vi "웹서버 수정 버전 1.vi"() -> ()   [LabVIEW 2019]
uses:
  <vilib>/httpClient/ClientHandle.ctl
  <vilib>/DAQmx/read.llb/DAQmx Read (Digital 1D Bool NChan 1Samp 1Line).vi
  <vilib>/DAQmx/read.llb/DAQmx Read (Analog 1D DBL 1Chan NSamp).vi
  <vilib>/Analysis/baseanly.llb/Mean (DBL).vi
  <vilib>/DAQmx/create/channels.llb/DAQmx Create Channel (DI-Digital Input).vi
  <vilib>/DAQmx/configure/timing.llb/DAQmx Timing (Sample Clock).vi
  <vilib>/DAQmx/create/channels.llb/DAQmx Create Channel (AI-Temperature-Thermocouple).vi
  <vilib>/httpClient/PUTBuffer.vi
  <vilib>/DAQmx/miscellaneous.llb/DAQmx Fill In Error Info.vi
  <vilib>/httpClient/LabVIEWHTTPClient.lvlib
  <vilib>/Analysis/NI_AALBase.lvlib
panel:
  out "y 3":u32
  out "y 2":u32
  out "F포맷 문자열":string[](array[string])
  out "data":bool[](array[boolean]) caption="데이터"
  out "headers 4":string caption="연결확인 메세지 출력"
  out "body 4":string caption="웹서버에 입력된 문자열"
  out "참조 번호 출력 2":T1 caption="client handle out"
  out "10진수 문자열":string[](array[string])
  in  "정지 2":bool
  in  "lines":tag caption="라인"
  in  "thermocouple type":i32(ring)=10072 caption="열전쌍 타입" items=["J"=10072, "K"=10073, "N"=10077, "R"=10082, "S"=10085, "T"=10086, "B"=10047, "E"=10055]
  in  "physical channels":tag caption="물리적 채널"
  out "숫자형":i32
  in  "불리언":bool
  out "y":u32
  out "headers 3":string caption="연결확인 메세지 출력"
  out "body 3":string caption="웹서버에 입력된 문자열"
  in  "참조 번호 입력":T1 caption="client handle out"
  out "참조 번호 출력":T1 caption="client handle out"
  out "error out":errorcluster caption="에러 출력"
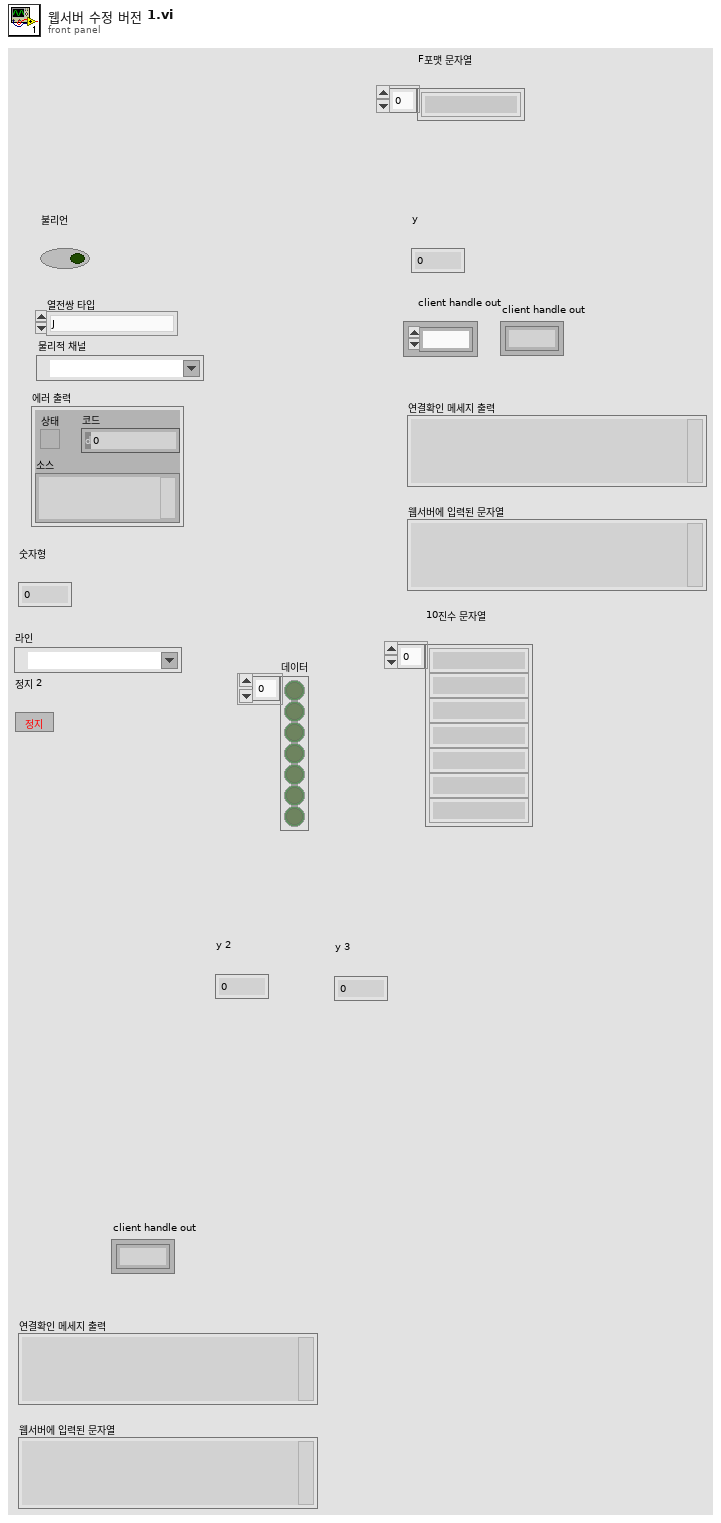
[diagram p1: front panel]
types:
  T1 = typedef "LabVIEWHTTPClient.lvlib/ClientHandle.ctl" = refnum<k1>
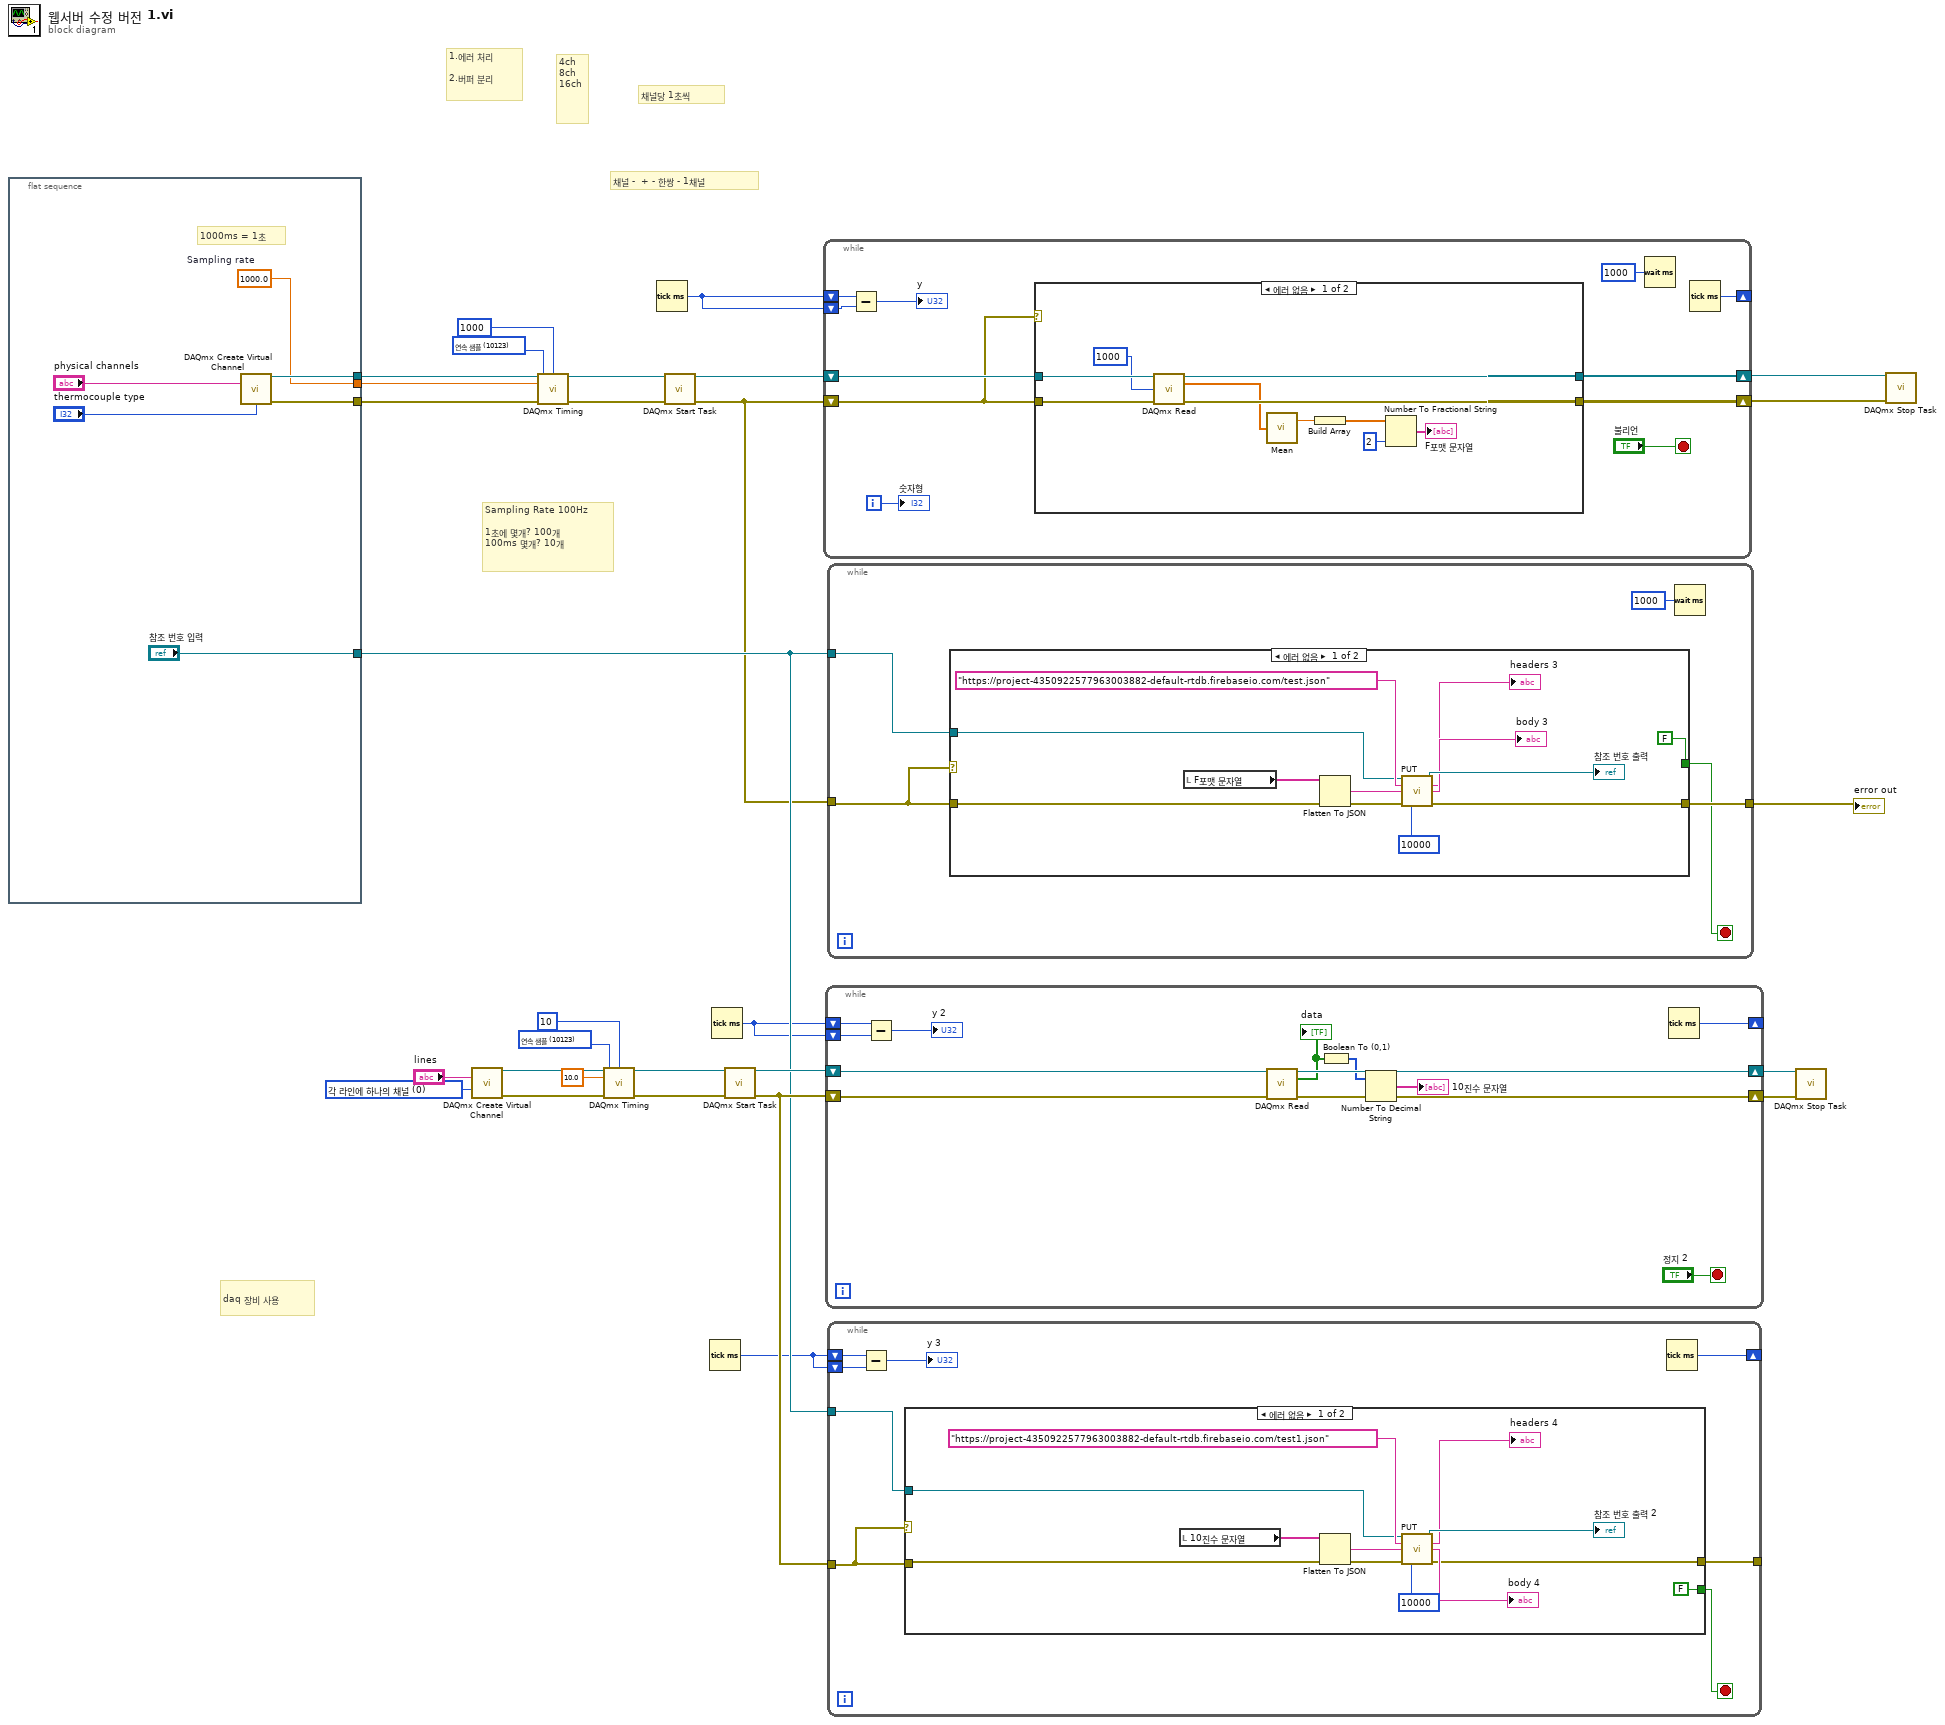
[diagram p0: block diagram]
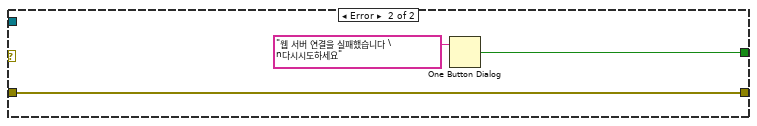
[diagram p2: hidden frame]
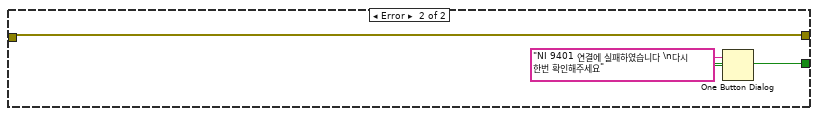
[diagram p4: hidden frame]
diagram:
  w20 = 10123 items=["유한 샘플"=10178, "연속 샘플"=10123, "하드웨어 타이밍에 의한 단일 포인트"=12522] ("sample mode")
  w21 = 0 items=["각 라인에 하나의 채널", "모든 라인에 하나의 채널"] ("line grouping")
  w23 = 10123 items=["유한 샘플"=10178, "연속 샘플"=10123, "하드웨어 타이밍에 의한 단일 포인트"=12522] ("sample mode")
  # "daq 장비 사용"
  # "1.에러 처리 \n\n2.버퍼 분리"
  # "채널 -  + - 한쌍 - 1채널"
  # "채널당 1초씩"
  # "4ch\n8ch\n16ch"
  # "Sampling Rate 100Hz\n\n1초에 몇개? 100개\n100ms 몇개? 10개"
  n1 = flat-sequence {
    tunnel: [w33] -> w29
    tunnel: [w32] -> w27
    tunnel: [w31] -> w24
    tunnel: ["참조 번호 입력"] -> w14
    frame #0 {
      w31 = 1000.0  # Sampling rate
      # "1000ms = 1초"
      n2 = call-poly <vilib>:"DAQmx Create Virtual Channel.vi"("physical channels"="physical channels", "thermocouple type"="thermocouple type") -> ("task out"=w33:refnum<k21>, "error out"=w32:errorcluster)  [unwired: 12 in]
    }
  }
  n3 = call-poly <vilib>:"DAQmx Create Virtual Channel.vi"("lines"="lines", "line grouping"=w21) -> ("task out"=w1:refnum<k21>, "error out"=w18:errorcluster)  [unwired: 12 in]
  n4 = call-poly <vilib>:"DAQmx Timing.vi"("task/channels in"=w29, "sample mode"=w23, "samples per channel"=1000, "rate"=w24, "error in"=w27) -> ("task out"=w28:refnum<k21>, "error out"=w26:errorcluster)  [unwired: 9 in]
  n5 = call-poly <vilib>:"DAQmx Timing.vi"("task/channels in"=w1, "sample mode"=w20, "samples per channel"=10, "rate"=10.0, "error in"=w18) -> ("task out"=w17:refnum<k21>, "error out"=w16:errorcluster)  [unwired: 9 in]
  n6 = Tick Count (ms)() -> (millisecond timer value=w6:u32)
  n7 = call <vilib>:"DAQmx Start Task.vi"("task/channels in"=w28, "error in"=w26) -> ("task out"=w7:refnum<k21>, "error out"=w5:errorcluster)  [unwired: 12 in]
  n8 = Tick Count (ms)() -> (millisecond timer value=w2:u32)
  n9 = Tick Count (ms)() -> (millisecond timer value=w3:u32)
  n10 = call <vilib>:"DAQmx Start Task.vi"("task/channels in"=w17, "error in"=w16) -> ("task out"=w22:refnum<k21>, "error out"=w15:errorcluster)  [unwired: 12 in]
  n11 = while {
    shift-right: [w45] -> w9
    shift-left: w7 -> [w46]
    shift-right: [w44] -> w8
    shift-left: w5 -> [w36]
    shift-right: [w41] -> _
    shift-left: w6 -> [w40]
    shift-left: w6 -> [w39]
    i -> [w43]
    stop <- "불리언" stop-if-true
    n12 = Subtract(x=w40, y=w39) -> (x-y=→"y":u32)
    n13 = case shown="에러 없음" w36 {
      tunnel: w46 -> [w56 w58]
      tunnel: w36 -> [w55 w57]
      tunnel: [w54 w58] -> w45
      tunnel: [w53 w57] -> w44
      frame No Error {
        n14 = call-poly <vilib>:"DAQmx Read.vi"("task/channels in"=w56, "number of samples per channel"=1000, "error in"=w55) -> ("task out"=w54:refnum<k21>, "data"=w49:dbl[], "error out"=w53:errorcluster)  [unwired: 10 in]
        n15 = call-poly <vilib>:"Mean.vi"("X"=w49) -> ("mean"=w48:dbl)  [unwired: 1 out]
        n16 = Build Array(w48) -> (w51:dbl[])
        n17 = Number To Fractional String(number=w51, precision (6)=i16 2 ("정밀도(6)")) -> (F-format string=→"F포맷 문자열":string[])  [unwired: 2 in]
      }
      frame Error {
        # "에러 발생시 재 연결 실시"
      }
    }
    n18 = Wait (ms)(milliseconds to wait=u32 1000 ("대기 시간 (ms)")) -> ()  [unwired: 1 out]
    n19 = Tick Count (ms)() -> (millisecond timer value=w41:u32)
    "숫자형" <- w43
  }
  n20 = while {
    shift-right: [w68] -> w12
    shift-left: w22 -> [w70]
    shift-right: [w67] -> w11
    shift-left: w15 -> [w69]
    shift-right: [w59] -> _
    shift-left: w3 -> [w61]
    shift-left: w3 -> [w60]
    stop <- "정지 2" stop-if-true
    n21 = Subtract(x=w61, y=w60) -> (x-y=→"y 2":u32)
    n22 = call-poly <vilib>:"DAQmx Read.vi"("task/channels in"=w70, "error in"=w69) -> ("task out"=w68:refnum<k21>, "data"=w64:bool[], "error out"=w67:errorcluster)  [unwired: 11 in]
    "data" <- w64
    n23 = Boolean To (0,1)(Boolean=w64) -> (0, 1=w63:i16[])
    n24 = Number To Decimal String(number=w63) -> (decimal integer string=→"10진수 문자열":string[])  [unwired: 1 in]
    n25 = Tick Count (ms)() -> (millisecond timer value=w59:u32)
  }
  n26 = while {
    tunnel: w5 -> [w72]
    tunnel: w14 -> [w74]
    tunnel: [w73] -> w4
    stop <- w71 stop-if-true
    n27 = case shown="에러 없음" w72 {
      tunnel: w72 -> [w80 w89]
      tunnel: w74 -> [w79 _]
      tunnel: [w78 w89] -> w73
      tunnel: [FALSE ("true") w88] -> w71
      frame No Error {
        n28 = local read "F포맷 문자열"() -> (w77:string[])
        n29 = Flatten To JSON(anything=w77, error in (no error)=w80) -> (JSON string=w84:string, 11:w83:errorcluster)  [unwired: 1 in]
        n30 = call-poly <vilib>:"PUT.vi"("client handle"=w79, "url"="https://project-4350922577963003882-default-rtdb.firebaseio.com/test.json", "buffer"=w84, "error in (no error)"=w83, "timeout (10000)"=10000) -> ("client handle out"=→"참조 번호 출력":T1, "headers"=→"headers 3":string, "body"=→"body 3":string, "error out"=w78:errorcluster)  [unwired: 7 in]
      }
      frame Error {
        n31 = One Button Dialog(message="웹 서버 연결을 실패했습니다 \n다시시도하세요" ("메시지")) -> (true=w88:bool)  [unwired: 1 in]
      }
    }
    n32 = Wait (ms)(milliseconds to wait=u32 1000 ("대기 시간 (ms)")) -> ()  [unwired: 1 out]
  }
  "error out" <- w4
  n33 = while {
    tunnel: w14 -> [w98]
    tunnel: [w97] -> _
    tunnel: w15 -> [w96]
    shift-right: [w94] -> _
    shift-left: w2 -> [w92]
    shift-left: w2 -> [w91]
    stop <- w95 stop-if-true
    n34 = Subtract(x=w92, y=w91) -> (x-y=→"y 3":u32)
    n35 = case shown="에러 없음" w96 {
      tunnel: w96 -> [w103 w112]
      tunnel: w98 -> [w100 _]
      tunnel: [w101 w112] -> w97
      tunnel: [FALSE ("true") w111] -> w95
      frame No Error {
        n36 = local read "10진수 문자열"() -> (w102:string[])
        n37 = Flatten To JSON(anything=w102, error in (no error)=w103) -> (JSON string=w107:string, 11:w106:errorcluster)  [unwired: 1 in]
        n38 = call-poly <vilib>:"PUT.vi"("client handle"=w100, "url"="https://project-4350922577963003882-default-rtdb.firebaseio.com/test1.json", "buffer"=w107, "error in (no error)"=w106, "timeout (10000)"=10000) -> ("client handle out"=→"참조 번호 출력 2":T1, "headers"=→"headers 4":string, "body"=→"body 4":string, "error out"=w101:errorcluster)  [unwired: 7 in]
      }
      frame Error {
        n39 = One Button Dialog(message="NI 9401 연결에 실패하였습니다 \n다시 한번 확인해주세요" ("메시지")) -> (true=w111:bool)  [unwired: 1 in]
      }
    }
    n40 = Tick Count (ms)() -> (millisecond timer value=w94:u32)
  }
  n41 = call <vilib>:"DAQmx Stop Task.vi"("task/channels in"=w12, "error in"=w11) -> ()  [unwired: 12 in, 2 out]
  n42 = call <vilib>:"DAQmx Stop Task.vi"("task/channels in"=w9, "error in"=w8) -> ()  [unwired: 12 in, 2 out]
